vi "Maxi Gauge suppress warning.vi"(1 "error in":errorcluster) -> (0 "error out":errorcluster)   [LabVIEW 2018, in "Maxi Gauge.lvlib"]
uses:
  Maxi Gauge.lvlib
panel:
  # "suppress warning #d1073676294"
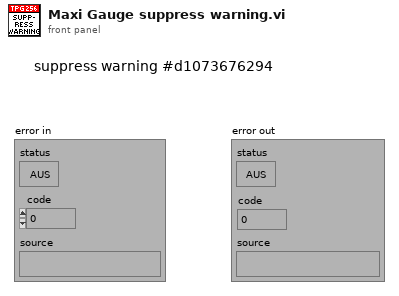
[diagram p1: front panel]
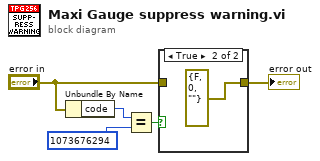
[diagram p0: block diagram]
diagram:
  n1 = Unbundle By Name("error in") -> ("code"=w2:i32)
  n2 = Equal?(x=w2, y=1073676294) -> (x = y?=w3:bool)
  n3 = case shown="True" w3 {
    tunnel: "error in" -> [w6 _]
    tunnel: [w6 cluster{bool, i32, "VI Name":string} {FALSE, 0, "VI Name"=""}] -> w4
    frame False {
    }
    frame True {
    }
  }
  "error out" <- w4
